vi "Weather data mabager.vi"(8 "umidade in":string, 9 "temperatura in":string, 10 "pressao in":string, 11 "Default Met":bool) -> (0 "umidade out":string, 1 "temperatura out":string, 2 "pressao out":string, 3 "weatherDefault":T1 caption="Dados meteorológicos default", 4 "led on":bool, 5 "wather160 led state":cluster{u32, u32}[](array[cluster]), 6 "valid file":bool, 7 "blink":bool)   [LabVIEW 2018]
uses:
  Global_Telescopio.vi
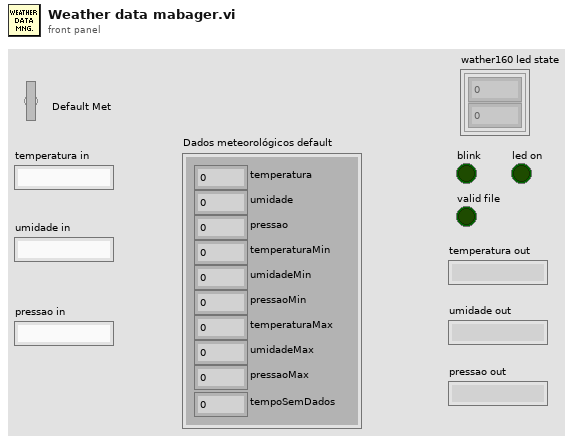
[diagram p1: front panel]
types:
  T1 = cluster{"temperatura":dbl, "umidade":dbl, "pressao":dbl, "temperaturaMin":dbl, "umidadeMin":dbl, "pressaoMin":dbl, "temperaturaMax":dbl, "umidadeMax":dbl, "pressaoMax":dbl, "tempoSemDados":dbl}
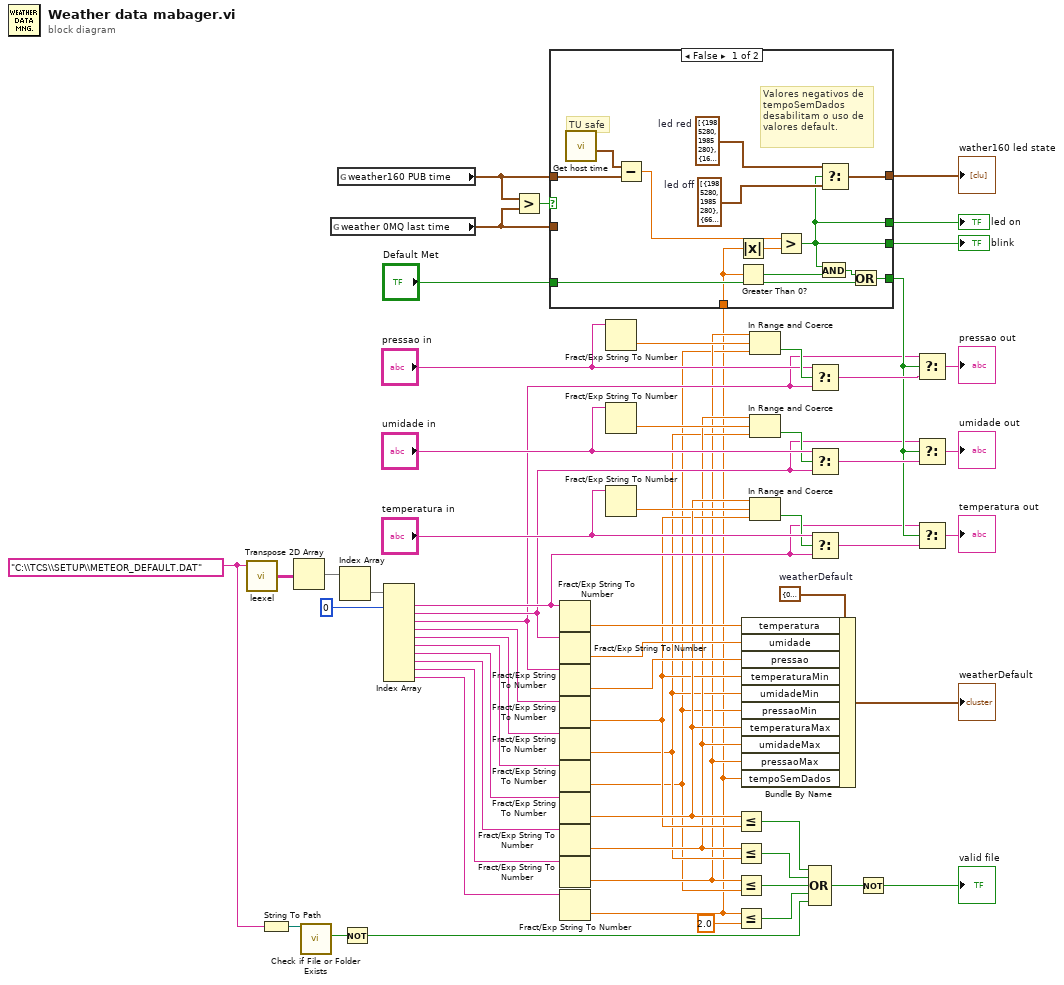
[diagram p0: block diagram]
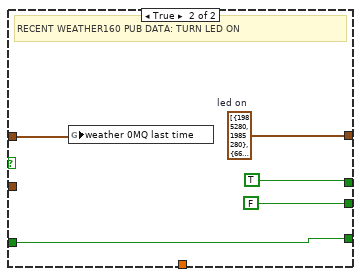
[diagram p2: hidden frame]
diagram:
  w48 = T1 {"temperatura"=0.0, "umidade"=0.0, "pressao"=0.0, "temperaturaMin"=0.0, "umidadeMin"=0.0, "pressaoMin"=0.0, "temperaturaMax"=0.0, "umidadeMax"=0.0, "pressaoMax"=0.0, "tempoSemDados"=0.0}  # weatherDefault
  w17 = "C:\\TCS\\SETUP\\METEOR_DEFAULT.DAT"
  n1 = call "leexel.vi"("path"=w17) -> ("array 5"=w60:string[][])  [unwired: 4 in]
  n2 = String To Path(string=w17) -> (path=w18:path)
  n3 = Transpose 2D Array(2D array=w60) -> (transposed array=w59:string[][])
  n4 = call <vilib>:"Check if File or Folder Exists.vi"("path"=w18) -> ("file or folder exists?"=w16:bool)  [unwired: 8 in, 2 out]
  n5 = global read "Global_Telescopio.vi" "weather 0MQ last time"() -> (w29:timestamp)
  n6 = global read "Global_Telescopio.vi" "weather160 PUB time"() -> (w28:timestamp)
  n7 = Index Array(array=w59) -> (element=w58:string[])  [unwired: 2 in]
  n8 = Not(x=w16) -> (.not. x?=w5:bool)
  n9 = Index Array(array=w58, index #1=0 ("index")) -> (element #1=w24:string, element #2=w23:string, element #3=w22:string, element #4=w30:string, element #5=w53:string, element #6=w52:string, element #7=w51:string, element #8=w50:string, element #9=w49:string, element #10=w46:string)  [unwired: 9 in]
  n10 = Greater?(x=w28, y=w29) -> (0:w27:bool)
  n11 = Fract/Exp String To Number(string=w24) -> (number=w56:dbl)  [unwired: 3 in, 1 out]
  n12 = Fract/Exp String To Number(string=w23) -> (number=w55:dbl)  [unwired: 3 in, 1 out]
  n13 = Fract/Exp String To Number(string=w22) -> (number=w54:dbl)  [unwired: 3 in, 1 out]
  n14 = Fract/Exp String To Number(string=w30) -> (number=w11:dbl)  [unwired: 3 in, 1 out]
  n15 = Fract/Exp String To Number(string=w53) -> (number=w9:dbl)  [unwired: 3 in, 1 out]
  n16 = Fract/Exp String To Number(string=w52) -> (number=w7:dbl)  [unwired: 3 in, 1 out]
  n17 = Fract/Exp String To Number(string=w51) -> (number=w12:dbl)  [unwired: 3 in, 1 out]
  n18 = Fract/Exp String To Number(string=w50) -> (number=w10:dbl)  [unwired: 3 in, 1 out]
  n19 = Fract/Exp String To Number(string=w49) -> (number=w8:dbl)  [unwired: 3 in, 1 out]
  n20 = Fract/Exp String To Number(string=w46) -> (number=w6:dbl)  [unwired: 3 in, 1 out]
  n21 = case shown="False" w27 {
    tunnel: w28 -> [w73 w77]
    tunnel: w29 -> [_ _]
    tunnel: [w71 w78] -> w21
    tunnel: w6 -> [w68 _]
    tunnel: "Default Met" -> [w70 w76]
    tunnel: [w67 w76] -> w25
    tunnel: [w62 FALSE] -> w19
    tunnel: [w62 TRUE] -> w20
    frame False {
      w72 = cluster{u32, u32}[] [{1985280, 1985280}, {16711680, 16711680}, {1985280, 1985280}, {6618880, 6618880}]  # led red
      w64 = cluster{u32, u32}[] [{1985280, 1985280}, {6618880, 6618880}, {1985280, 1985280}, {6618880, 6618880}]  # led off
      # "TU safe"
      # "Valores negativos de\ntempoSemDados \ndesabilitam o uso de\nvalores default."
      n22 = call "Get host time.vi"() -> ("BR current time"=w61:timestamp)  [unwired: 8 in, 3 out]
      n23 = Subtract(x=w61, y=w73) -> (x-y=w65:dbl)
      n24 = Absolute Value(x=w68) -> (abs(x)=w69:dbl)
      n25 = Greater Than 0?(x=w68) -> (x > 0?=w66:bool)
      n26 = Greater?(x=w65, y=w69) -> (0:w62:bool)
      n27 = And(x=w62, y=w66) -> (x .and. y?=w63:bool)
      n28 = Select(t=w72, s=w62, f=w64) -> (s? t:f=w71:cluster{u32, u32}[])
      n29 = Or(x=w63, y=w70) -> (x .or. y?=w67:bool)
    }
    frame True {
      w78 = cluster{u32, u32}[] [{1985280, 1985280}, {6618880, 6618880}, {1985280, 1985280}, {6618880, 6618880}]  # led on
      # "RECENT WEATHER160 PUB DATA: TURN LED ON"
      n30 = global write "Global_Telescopio.vi" "weather 0MQ last time"(w77) -> ()
    }
  }
  "led on" <- w20
  "blink" <- w19
  "wather160 led state" <- w21
  n31 = Fract/Exp String To Number(string="pressao in") -> (number=w44:dbl)  [unwired: 3 in, 1 out]
  n32 = Fract/Exp String To Number(string="umidade in") -> (number=w43:dbl)  [unwired: 3 in, 1 out]
  n33 = Fract/Exp String To Number(string="temperatura in") -> (number=w42:dbl)  [unwired: 3 in, 1 out]
  n34 = Less Or Equal?(x=w12, y=w11) -> (x <= y?=w13:bool)
  n35 = Less Or Equal?(x=w10, y=w9) -> (x <= y?=w14:bool)
  n36 = Less Or Equal?(x=w8, y=w7) -> (x <= y?=w15:bool)
  n37 = Less Or Equal?(x=w6, y=2.0) -> (x <= y?=w3:bool)
  n38 = Bundle By Name(cluster=w48, "temperatura"=w56, "umidade"=w55, "pressao"=w54, "temperaturaMin"=w11, "umidadeMin"=w9, "pressaoMin"=w7, "temperaturaMax"=w12, "umidadeMax"=w10, "pressaoMax"=w8, "tempoSemDados"=w6) -> (→"weatherDefault":T1)
  n39 = In Range and Coerce(upper limit=w8, x=w44, lower limit=w7) -> (In Range?=w37:bool)  [unwired: 1 out]
  n40 = In Range and Coerce(upper limit=w10, x=w43, lower limit=w9) -> (In Range?=w38:bool)  [unwired: 1 out]
  n41 = In Range and Coerce(upper limit=w12, x=w42, lower limit=w11) -> (In Range?=w41:bool)  [unwired: 1 out]
  n42 = Compound Arithmetic op=OR(w13, w14, w15, w3, w5) -> (w2:bool)
  n43 = Select(t="pressao in", s=w37, f=w22) -> (s? t:f=w36:string)
  n44 = Select(t="umidade in", s=w38, f=w23) -> (s? t:f=w35:string)
  n45 = Select(t="temperatura in", s=w41, f=w24) -> (s? t:f=w40:string)
  n46 = Not(x=w2) -> (.not. x?=→"valid file":bool)
  n47 = Select(t=w22, s=w25, f=w36) -> (s? t:f=→"pressao out":string)
  n48 = Select(t=w23, s=w25, f=w35) -> (s? t:f=→"umidade out":string)
  n49 = Select(t=w24, s=w25, f=w40) -> (s? t:f=→"temperatura out":string)
